vi "Stimuli_Widefield.vi"() -> ()   [LabVIEW 2014]
uses:
  Widefield_globals.vi
  Instance           7 17Saved   load_save .vi
  Instance          10 17Saved   load_save .vi
  <vilib>/Utility/file.llb/Write To Spreadsheet File (I64).vi
  <vilib>/Utility/file.llb/Read From Spreadsheet File (DBL).vi
  Instance           4 17Saved   load_save .vi
panel:
  in  "Clear":bool
  in  "Stop:":i32
  in  "Copy Row1":bool
  in  "Increment":i32
  in  "Start:":i32
  in  "Frame Calculator":bool
  out "Frames":i32
  in  "Time (s)":dbl
  out "Current Frame rate (Hz)":i32
  in  "Save":bool
  in  "StimulusTable":string[][](table)
  out "# Odors":i32
  in  "Done!":bool
  in  "Set Sequence":bool
  in  "Load Experiment":bool
  # "ODOR IDs: Isoamyl acetate (7); ethyl tiglate (8); Ethyl butyrate (9); hexanal (10); 2,3 pentanedione (11);"
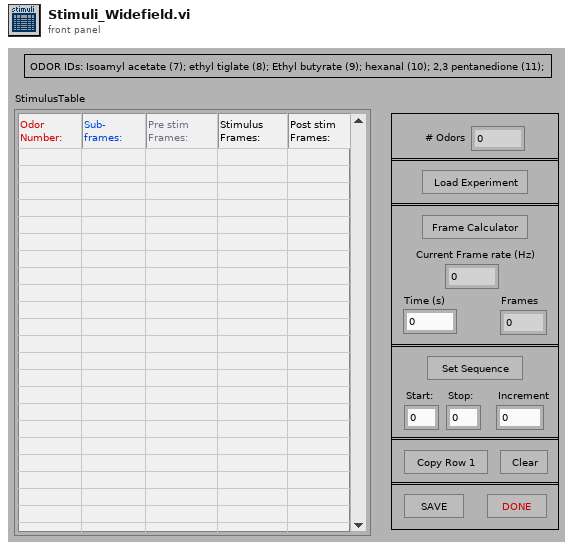
[diagram p1: front panel]
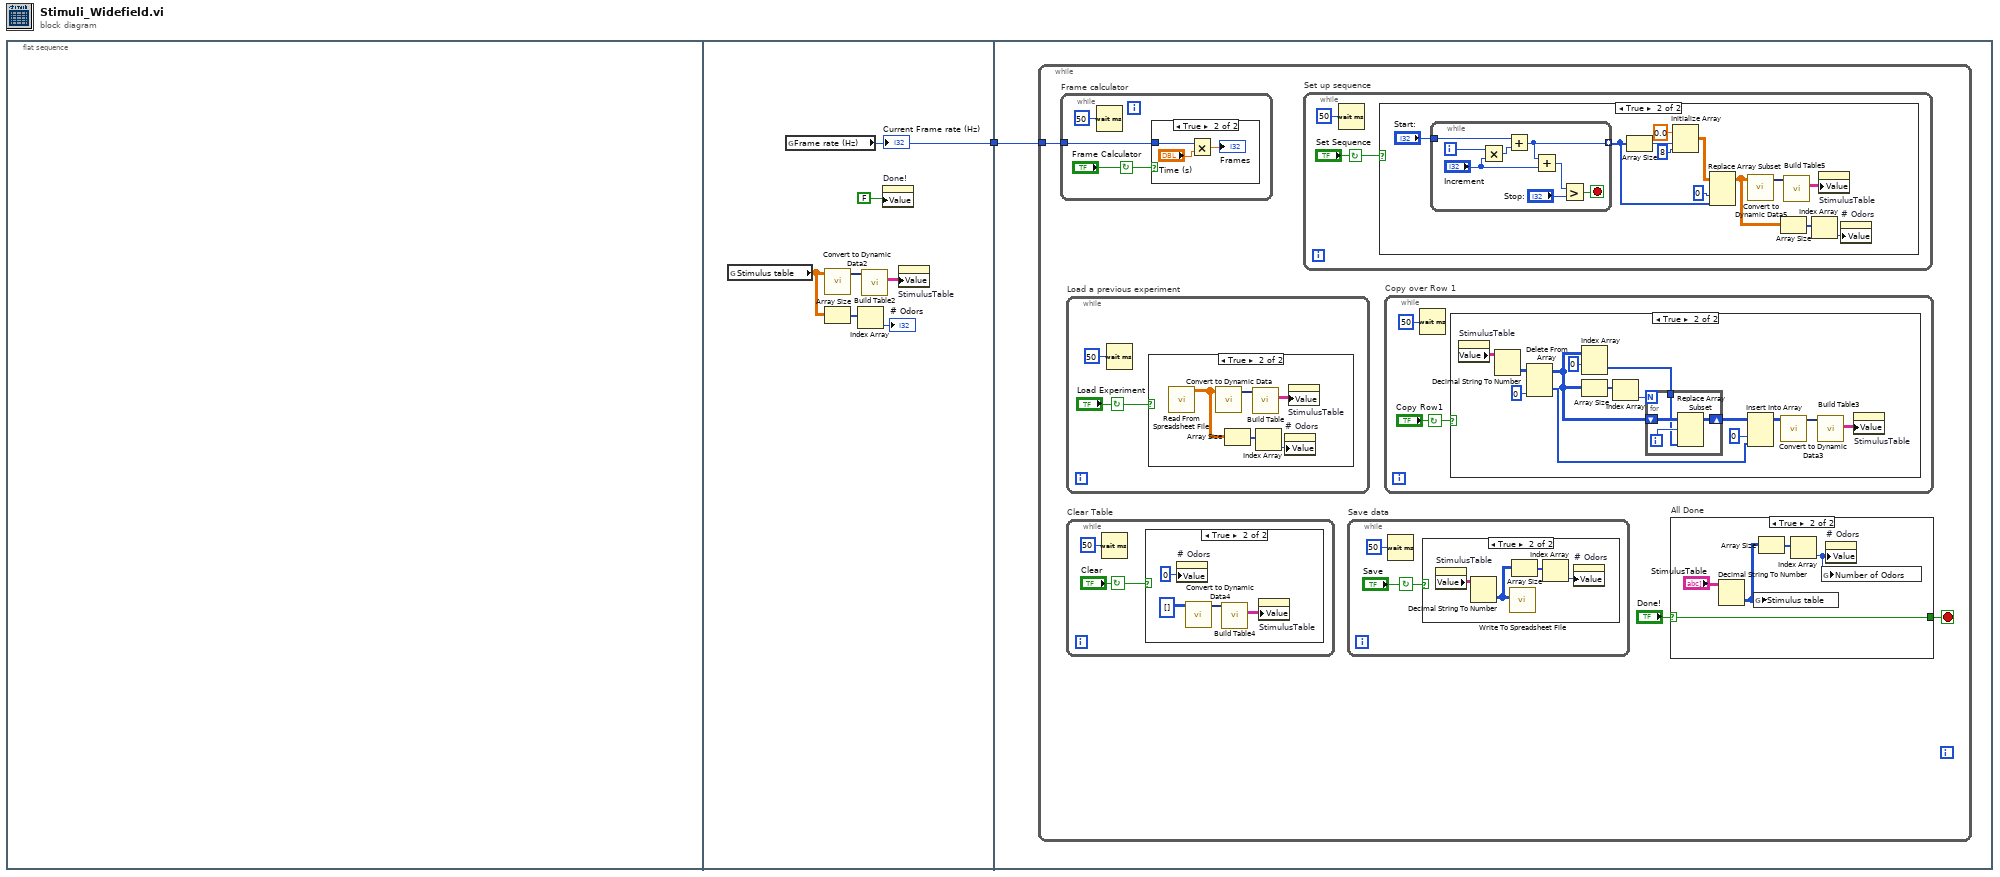
[diagram p0: block diagram]
diagram:
  n1 = flat-sequence {
    tunnel: [w6] -> w1
    tunnel: w1 -> [w9]
    frame #0 {
    }
    frame #1 {
      n2 = global read "Widefield_globals.vi" "Stimulus table"() -> (w4:dbl[][])
      n3 = global read "Widefield_globals.vi" "Frame rate (Hz)"() -> (w6:u16)
      "Current Frame rate (Hz)" <- w6
      n4 = call "Convert to Dynamic Data2"("2D Array"=w4) -> ("Dynamic Data Type"=w8:dynamicdata)  [unwired: 3 out]
      n5 = Array Size(array=w4) -> (size(s)=w7:i32[])
      n6 = Index Array(array=w7) -> (element=→"# Odors":i32)  [unwired: 1 in]
      n7 = call "Build Table2"("Signals"=w8) -> ("Table"=w2:string[][])  [unwired: 4 in, 6 out]
      n8 = property on="Done!" class="Bool (strict)"("Value"=FALSE ("Done!")) -> ()  [unwired: 2 in, 2 out]
      n9 = property on="StimulusTable" class="Tbl (strict)"("Value"=w2) -> ()  [unwired: 2 in, 2 out]
    }
    frame #2 {
      n10 = while {
        tunnel: w9 -> [w11]
        stop <- w10 stop-if-true
        n11 = while "Frame calculator" {
          tunnel: w11 -> [w49]
          stop <- "Frame Calculator" continue-if-true
          n12 = Wait (ms)(milliseconds to wait=50) -> ()  [unwired: 1 out]
          n13 = case shown="True" "Frame Calculator" {
            tunnel: w49 -> [_ w53]
            frame False {
            }
            frame True {
              n14 = Multiply(x=w53, y="Time (s)") -> (x*y=→"Frames":dbl)
            }
          }
        }
        n15 = while "Load a previous experiment" {
          stop <- "Load Experiment" continue-if-true
          n16 = Wait (ms)(milliseconds to wait=50) -> ()  [unwired: 1 out]
          n17 = case shown="True" "Load Experiment" {
            frame False {
            }
            frame True {
              n18 = call-poly <vilib>:"Read From Spreadsheet File.vi"() -> ("all rows"=w19:dbl[][])  [unwired: 4 in, 7 out]
              n19 = call "Convert to Dynamic Data"("2D Array"=w19) -> ("Dynamic Data Type"=w18:dynamicdata)  [unwired: 3 out]
              n20 = Array Size(array=w19) -> (size(s)=w17:i32[])
              n21 = call "Build Table"("Signals"=w18) -> ("Table"=w16:string[][])  [unwired: 4 in, 6 out]
              n22 = Index Array(array=w17) -> (element=w15:i32)  [unwired: 1 in]
              n23 = property on="# Odors" class="DigNum (strict)"("Value"=w15) -> ()  [unwired: 2 in, 2 out]
              n24 = property on="StimulusTable" class="Tbl (strict)"("Value"=w16) -> ()  [unwired: 2 in, 2 out]
            }
          }
        }
        n25 = while "Clear Table" {
          stop <- "Clear" continue-if-true
          n26 = Wait (ms)(milliseconds to wait=50) -> ()  [unwired: 1 out]
          n27 = case shown="True" "Clear" {
            frame False {
            }
            frame True {
              n28 = property on="# Odors" class="DigNum (strict)"("Value"=0 ("# Odors")) -> ()  [unwired: 2 in, 2 out]
              n29 = call "Convert to Dynamic Data4"("2D Array"=i32[][] []) -> ("Dynamic Data Type"=w24:dynamicdata)  [unwired: 3 out]
              n30 = call "Build Table4"("Signals"=w24) -> ("Table"=w25:string[][])  [unwired: 4 in, 6 out]
              n31 = property on="StimulusTable" class="Tbl (strict)"("Value"=w25) -> ()  [unwired: 2 in, 2 out]
            }
          }
        }
        n32 = while "Set up sequence" {
          stop <- "Set Sequence" continue-if-true
          n33 = Wait (ms)(milliseconds to wait=50) -> ()  [unwired: 1 out]
          n34 = case shown="True" "Set Sequence" {
            frame False {
            }
            frame True {
              n35 = while {
                tunnel: "Start:" -> [w47]
                tunnel: [w42] -> w33 mode=indexing
                i -> [w43]
                stop <- w45 stop-if-true
                n36 = Multiply(x=w43, y="Increment") -> (x*y=w46:i32)
                n37 = Add(x=w47, y=w46) -> (x+y=w42:i32)
                n38 = Add(x=w42, y="Increment") -> (x+y=w40:i32)
                n39 = Greater?(x=w40, y="Stop:") -> (0:w45:bool)
              }
              n40 = Array Size(array=w33) -> (size(s)=w38:i32)
              n41 = Initialize Array(0.0 ("element"), w38, 8 ("dimension size")) -> (w35:dbl[][])
              n42 = Replace Array Subset(array=w35, new element=w33, index (col)=0 ("disabled index (col)")) -> (w28:dbl[][])  [unwired: 1 in]
              n43 = call "Convert to Dynamic Data5"("2D Array"=w28) -> ("Dynamic Data Type"=w29:dynamicdata)  [unwired: 3 out]
              n44 = Array Size(array=w28) -> (size(s)=w30:i32[])
              n45 = call "Build Table5"("Signals"=w29) -> ("Table"=w31:string[][])  [unwired: 4 in, 6 out]
              n46 = Index Array(array=w30) -> (element=w32:i32)  [unwired: 1 in]
              n47 = property on="StimulusTable" class="Tbl (strict)"("Value"=w31) -> ()  [unwired: 2 in, 2 out]
              n48 = property on="# Odors" class="DigNum (strict)"("Value"=w32) -> ()  [unwired: 2 in, 2 out]
            }
          }
        }
        n49 = while "Save data" {
          stop <- "Save" continue-if-true
          n50 = Wait (ms)(milliseconds to wait=50) -> ()  [unwired: 1 out]
          n51 = case shown="True" "Save" {
            frame False {
            }
            frame True {
              n52 = property on="StimulusTable" class="Tbl (strict)"() -> ("Value"=w64:string[][])  [unwired: 2 in, 2 out]
              n53 = Decimal String To Number(string=w64) -> (number=w63:i32[][])  [unwired: 3 out]
              n54 = call-poly <vilib>:"Write To Spreadsheet File.vi"("2D data"=w63) -> ()  [unwired: 5 in, 3 out]
              n55 = Array Size(array=w63) -> (size(s)=w65:i32[])
              n56 = Index Array(array=w65) -> (element=w62:i32)  [unwired: 1 in]
              n57 = property on="# Odors" class="DigNum (strict)"("Value"=w62) -> ()  [unwired: 2 in, 2 out]
            }
          }
        }
        n58 = while "Copy over Row 1" {
          stop <- "Copy Row1" continue-if-true
          n59 = Wait (ms)(milliseconds to wait=50) -> ()  [unwired: 1 out]
          n60 = case shown="True" "Copy Row1" {
            frame False {
            }
            frame True {
              n61 = property on="StimulusTable" class="Tbl (strict)"() -> ("Value"=w81:string[][])  [unwired: 2 in, 2 out]
              n62 = Decimal String To Number(string=w81) -> (number=w69:i32[][])  [unwired: 3 out]
              n63 = Delete From Array(array=w69, index (col)=0 ("disabled index (col)")) -> (deleted portion=w78:i32[], array with subset deleted=w72:i32[][])  [unwired: 2 in]
              n64 = Index Array(array=w72, index (row)=0) -> (element=w75:i32[])  [unwired: 1 in]
              n65 = Array Size(array=w72) -> (size(s)=w73:i32[])
              n66 = Index Array(array=w73) -> (element=w74:i32)  [unwired: 1 in]
              n67 = for {
                N: w74 -> [_]
                shift-right: [w84] -> w76
                shift-left: w72 -> [w85]
                tunnel: w75 -> [w82]
                i -> [w83]
                n68 = Replace Array Subset(array=w85, new element=w82, index (row)=w83) -> (w84:i32[][])  [unwired: 1 in]
              }
              n69 = Insert Into Array(array=w76, index (col)=0 ("disabled index (col)"), new element=w78) -> (w68:i32[][])  [unwired: 1 in]
              n70 = call "Convert to Dynamic Data3"("2D Array"=w68) -> ("Dynamic Data Type"=w80:dynamicdata)  [unwired: 3 out]
              n71 = call "Build Table3"("Signals"=w80) -> ("Table"=w79:string[][])  [unwired: 4 in, 6 out]
              n72 = property on="StimulusTable" class="Tbl (strict)"("Value"=w79) -> ()  [unwired: 2 in, 2 out]
            }
          }
        }
        n73 = case "All Done" shown="True" "Done!" {
          selector: "Done!" -> [w54 w55]
          tunnel: [w54 w55] -> w10
          frame False {
          }
          frame True {
            n74 = Decimal String To Number(string="StimulusTable") -> (number=w58:i32[][])  [unwired: 3 out]
            n75 = global write "Widefield_globals.vi" "Stimulus table"(w58) -> ()
            n76 = Array Size(array=w58) -> (size(s)=w59:i32[])
            n77 = Index Array(array=w59) -> (element=w57:i32)  [unwired: 1 in]
            n78 = global write "Widefield_globals.vi" "Number of Odors"(w57) -> ()
            n79 = property on="# Odors" class="DigNum (strict)"("Value"=w57) -> ()  [unwired: 2 in, 2 out]
          }
        }
      }
    }
  }
